vi "LIN Laden Errors.vi"(8 "Fehler (Eingang, kein Fehler)":errorcluster, 11 "Ident Cluster":T1) -> (0 "error out":errorcluster, 1 "Error orccured":bool, 2 "LIN Loading Error Description Array":T2(array[cluster]), 3 "Ident Cluster out":T1, 4 "LIN Loading Errors Array":string[](array[string]))   [LabVIEW 2020, in "Linearisierung v2.lvlib" / "SpanEinstellungen.lvlib"]
uses:
  SpanEinstellungen.lvlib
  LIN Loading Errors.ctl
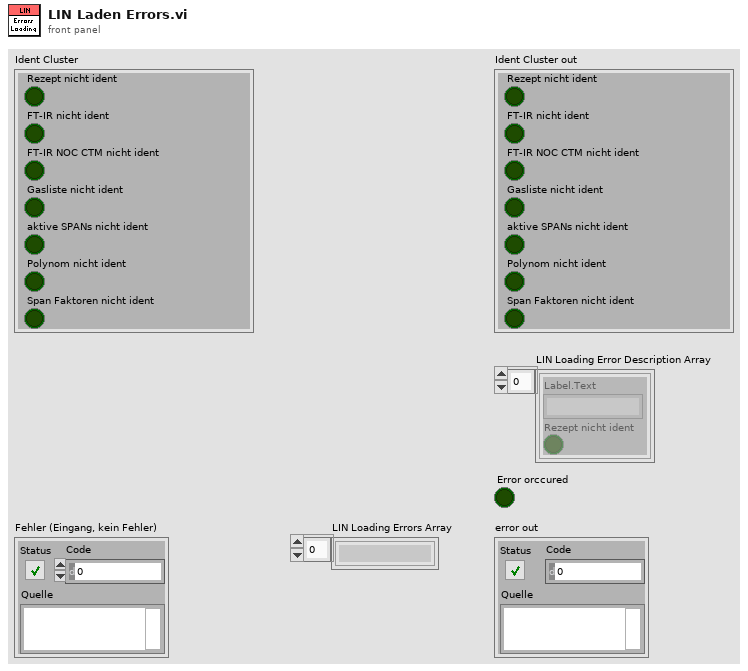
[diagram p1: front panel]
types:
  T1 = typedef "Linearisierung v2.lvlib/SpanEinstellungen.lvlib/LIN Loading Errors.ctl" = cluster{"Rezept nicht ident":bool, "FT-IR nicht ident":bool, "FT-IR NOC CTM nicht ident":bool, "Gasliste nicht ident":bool, "aktive SPANs nicht ident":bool, "Polynom nicht ident":bool, "Span Faktoren nicht ident":bool}
  T2 = cluster{"Label.Text":string, "Rezept nicht ident":bool}[]
  T3 = cluster{"Label.Text":string, "Rezept nicht ident":bool}
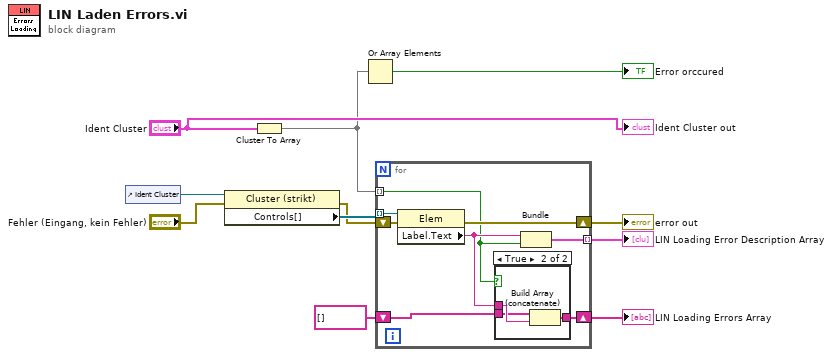
[diagram p0: block diagram]
diagram:
  n1 = control-ref of="Ident Cluster"() -> (w11:refnum<vi>)
  n2 = property class="Cluster (strikt)"(reference=w11, error in="Fehler (Eingang, kein Fehler)") -> (error out=w7:errorcluster, "Controls[]"=w10:refnum<vi>[])  [unwired: 1 out]
  n3 = Cluster To Array(cluster="Ident Cluster") -> (array=w4:bool[])
  n4 = Or Array Elements(Boolean array=w4) -> (logical OR=→"Error orccured":bool)
  n5 = for {
    tunnel: w10 -> [w19] mode=indexing
    shift-right: [w17] -> w6
    shift-left: w7 -> [w18]
    tunnel: w4 -> [w12] mode=indexing
    tunnel: [w16] -> w5 mode=indexing
    shift-right: [w14] -> w1
    shift-left: string[] [] -> [w13]
    n6 = property class="Elem"(reference=w19, error in=w18) -> (error out=w17:errorcluster, "Label.Text"=w15:string)  [unwired: 1 out]
    n7 = case shown="True" w12 {
      tunnel: w15 -> [_ w23]
      tunnel: [w20 w22] -> w14
      tunnel: w13 -> [w20 w21]
      frame False {
      }
      frame True {
        n8 = Build Array (concatenate)(w21, w23) -> (w22:string[])
      }
    }
    n9 = Bundle("Label.Text"=w15, "Rezept nicht ident"=w12) -> (w16:T3)  [unwired: 1 in]
  }
  "error out" <- w6
  "LIN Loading Error Description Array" <- w5
  "LIN Loading Errors Array" <- w1
  "Ident Cluster out" <- "Ident Cluster"
